vi "Move_pico.vi"(6 "Device Address In":i32, 7 "DeviceKey In":string, 8 "error in (no error)":errorcluster, 9 "CmdLib In":refnum<k24>, 10 "Relative Steps":i32, 11 "Motor #":i32=1) -> (0 "error out 2":errorcluster, 1 "CmdLib Out":refnum<k24>)   [LabVIEW 2014]
uses:
  C:/Program Files/New Focus/New Focus Picomotor Application/Samples/CmdLib.dll
  Program Files/New Focus/New Focus Picomotor Application/Samples/CmdLib.dll
panel:
  out "Position Status":i32
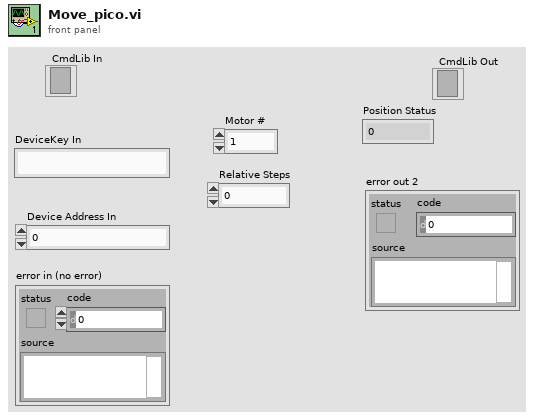
[diagram p1: front panel]
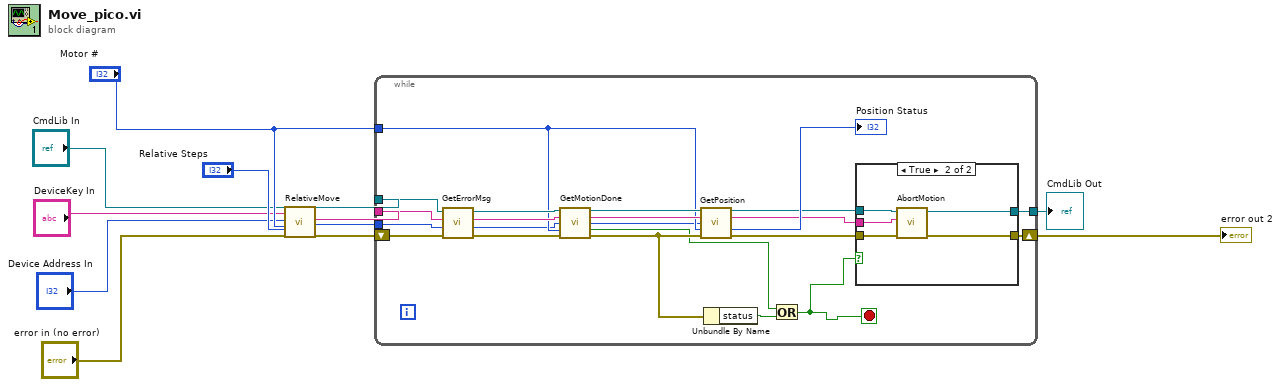
[diagram p0: block diagram]
diagram:
  n1 = call "RelativeMove.vi"("CmdLib In"="CmdLib In", "DeviceKey In"="DeviceKey In", "Device Address In"="Device Address In", "Motor"="Motor #", "Relative Steps"="Relative Steps", "error in (no error)"="error in (no error)") -> ("CmdLib Out"=w12:refnum<k24>, "DeviceKey Out"=w11:string, "Device Address Out"=w8:i32, "error out"=w10:errorcluster)  [unwired: 10 in]
  n2 = while {
    tunnel: "Motor #" -> [w30]
    tunnel: w12 -> [w29]
    tunnel: w11 -> [w28]
    tunnel: [w18] -> w6
    tunnel: w8 -> [w16]
    shift-right: [w20] -> w7
    shift-left: w10 -> [w27]
    stop <- w13 stop-if-true
    n3 = call "GetErrorMsg.vi"("error in (no error)"=w27, "Device Address In"=w16, "DeviceKey In"=w28, "CmdLib In"=w29) -> ("error out"=w26:errorcluster, "Device Address Out"=w15:i32, "DeviceKey Out"=w32:string, "CmdLib Out"=w31:refnum<k24>)
    n4 = call "GetMotionDone.vi"("CmdLib In"=w31, "DeviceKey In"=w32, "Device Address In"=w15, "Motor"=w30, "error in (no error)"=w26) -> ("CmdLib Out"=w33:refnum<k24>, "DeviceKey Out"=w34:string, "Device Address Out"=w14:i32, "Is Motion Done"=w23:bool, "error out"=w24:errorcluster)  [unwired: 6 in]
    n5 = call "GetPosition.vi"("CmdLib In"=w33, "DeviceKey In"=w34, "Device Address In"=w14, "Motor"=w30, "error in (no error)"=w24) -> ("CmdLib Out"=w19:refnum<k24>, "DeviceKey Out"=w17:string, "Position"=→"Position Status":i32, "error out"=w21:errorcluster)  [unwired: 6 in, 1 out]
    n6 = Unbundle By Name(w24) -> ("status"=w25:bool)
    n7 = Or(x=w23, y=w25) -> (x .or. y?=w13:bool)
    n8 = case shown="True" w13 {
      tunnel: w21 -> [w35 w41]
      tunnel: [w35 w40] -> w20
      tunnel: w19 -> [w36 w39]
      tunnel: [w36 w38] -> w18
      tunnel: w17 -> [_ w37]
      frame False {
      }
      frame True {
        n9 = call "AbortMotion.vi"("error in (no error)"=w41, "DeviceKey In"=w37, "CmdLib In"=w39) -> ("error out"=w40:errorcluster, "CmdLib Out"=w38:refnum<k24>)  [unwired: 1 in, 2 out]
      }
    }
  }
  "error out 2" <- w7
  "CmdLib Out" <- w6
